vi "tatrocki_target_C2.vi"   [LabVIEW 2020]
uses:
  <vilib>/platform/TimedLoop/XDataNode/XDataNode.xnode
  <vilib>/Platform/TimedLoop/XDataNode/nitl_modes.ctl
  <vilib>/Platform/TimedLoop/XDataNode/XDNodeRunTimeDep.lvlib
  <vilib>/Platform/TimedLoop/XDataNode/wakeup.ctl
  <vilib>/Platform/TimedLoop/XDataNode/timing_clust.ctl
types:
  T1 = typedef "XDNodeRunTimeDep.lvlib/timing_clust.ctl" = cluster{"Expected End [f-1]":u64, "Actual End [f-1]":u64, "Finished Late? [f-1]":bool, "Expected End [i-1]":u64, "Actual End [i-1]":u64, "Finished Late? [i-1]":bool, "Expected Start [i]":u64, "Actual Start [i]":u64, "Expected Start [f]":u64, "Actual Start [f]":u64, "Source Name":string, "Structure Name":string, "Period":i64, "Deadline":i64, "Offset":i64, "Start":i64, "Priority":i32, "Timeout":i32, "Mode":T2, "Wakeup Reason":T3, "Error":errorcluster, "Source Type":string, "Secondary Source Type":string, "Global End Time":u64, "Global Start Time":u64, "Frame Duration":u64, "Iteration Duration":u64, "Assigned CPU":i32, "I/O Scan Engine Mode":u32}
  T2 = typedef "XDNodeRunTimeDep.lvlib/nitl_modes.ctl" = enum32{"No Change", "Process missed periods, maintain original phase", "Discard missed periods, maintain original phase", "Process missed periods, ignore original phase", "Discard missed periods, ignore original phase"}
  T3 = typedef "XDNodeRunTimeDep.lvlib/wakeup.ctl" = enum32{"Normal", "Aborted", "Asynchronous wakeup", "Timing source error", "Timed loop error", "Timeout"}
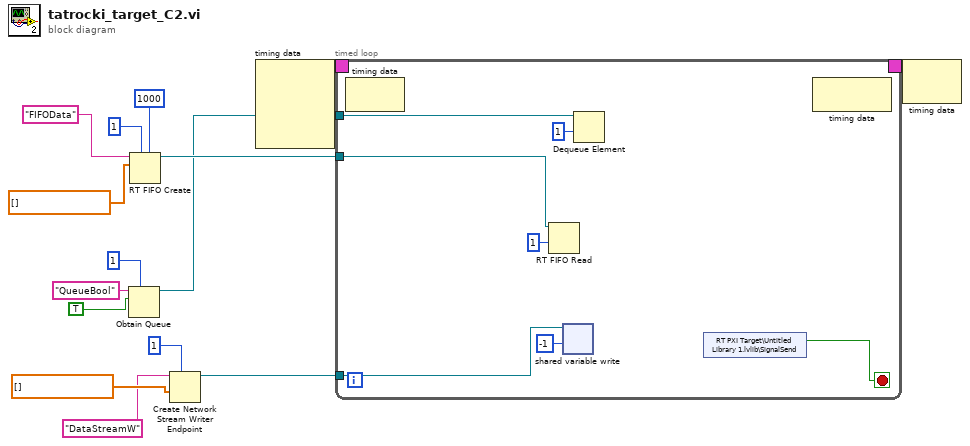
[diagram p0: block diagram]
diagram:
  n1 = Obtain Queue(max queue size (-1, unlimited)=1, name (unnamed)="QueueBool", element data type=TRUE) -> (queue out=w2:refnum<queue>)  [unwired: 2 in, 2 out]
  n2 = RT FIFO Create(0:"FIFOData" ("name (unnamed)"), 1:dbl[] [], 4:u32 1 ("size (10)"), 6:u32 1000 ("elements in array (1)")) -> (8:w3:refnum<k33>)  [unwired: 4 in, 2 out]
  n3 = Create Network Stream Writer Endpoint(7:1 ("writer buffer size"), 9:dbl[] [], 11:"DataStreamW" ("writer name")) -> (3:w1:refnum<k21>)  [unwired: 4 in, 1 out]
  n4 = node-c288() -> (w15:T1)  [unwired: 4 in]
  n5 = timed-loop {
    timing: w15 -> [_]
    timing-out: [_] -> w14
    tunnel: w3 -> [w22]
    tunnel: w2 -> [w21]
    tunnel: w1 -> [w20]
    stop <- w16 stop-if-true
    n6 = node-c288() -> ()  [unwired: 1 in, 1 out]
    n7 = RT FIFO Read(0:w22, 2:1 ("timeout in ms (0)")) -> ()  [unwired: 2 in, 5 out]
    n8 = shared-variable-write(w20, -1 ("timeout ms (-1)")) -> ()  [unwired: 2 in, 3 out]
    n9 = Dequeue Element(queue=w21, timeout in ms (-1)=1) -> ()  [unwired: 1 in, 4 out]
    n10 = shared-variable "RT PXI Target\\Untitled Library 1.lvlib\\SignalSend"() -> (w16:bool)  [unwired: 1 in, 1 out]
    n11 = node-c288() -> ()  [unwired: 1 in, 1 out]
  }
  n12 = node-c288(w14) -> ()  [unwired: 1 out]
